vi "CAN自动测试.vi"(10 "选择?":bool) -> ()   [LabVIEW 2010]
uses:
  全局量/试验配置信息.vi
  全局量/自动测试结果.vi
panel:
  in  "同步_2":i32
  in  "同步_1":i32
  out "结束?":bool
  in  "CAN_4_4":u16
  in  "CAN_4_3":u16
  in  "CAN_4_2":u16
  in  "CAN_4_1":u16
  in  "CAN_3_4":u16
  in  "CAN_3_3":u16
  in  "CAN_3_2":u16
  in  "CAN_3_1":u16
  in  "CAN_2_4":u16
  in  "CAN_2_3":u16
  in  "CAN_2_2":u16
  in  "CAN_2_1":u16
  in  "CAN_1_4":u16
  in  "CAN_1_3":u16
  in  "CAN_1_2":u16
  in  "CAN_1_1":u16
  # "CAN1"
  # "CAN2"
  # "CAN3"
  # "CAN4"
  # "测试结论："
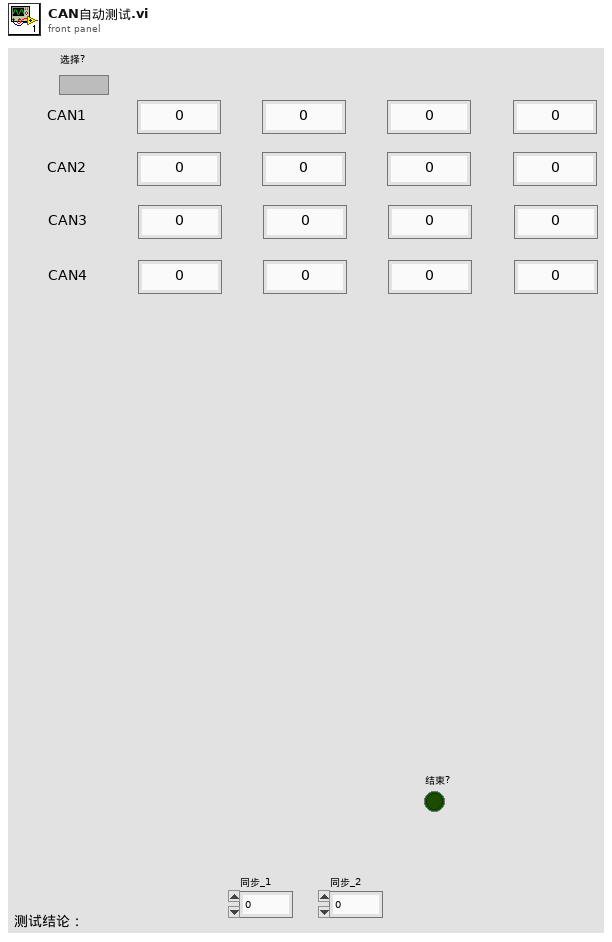
[diagram p1: front panel]
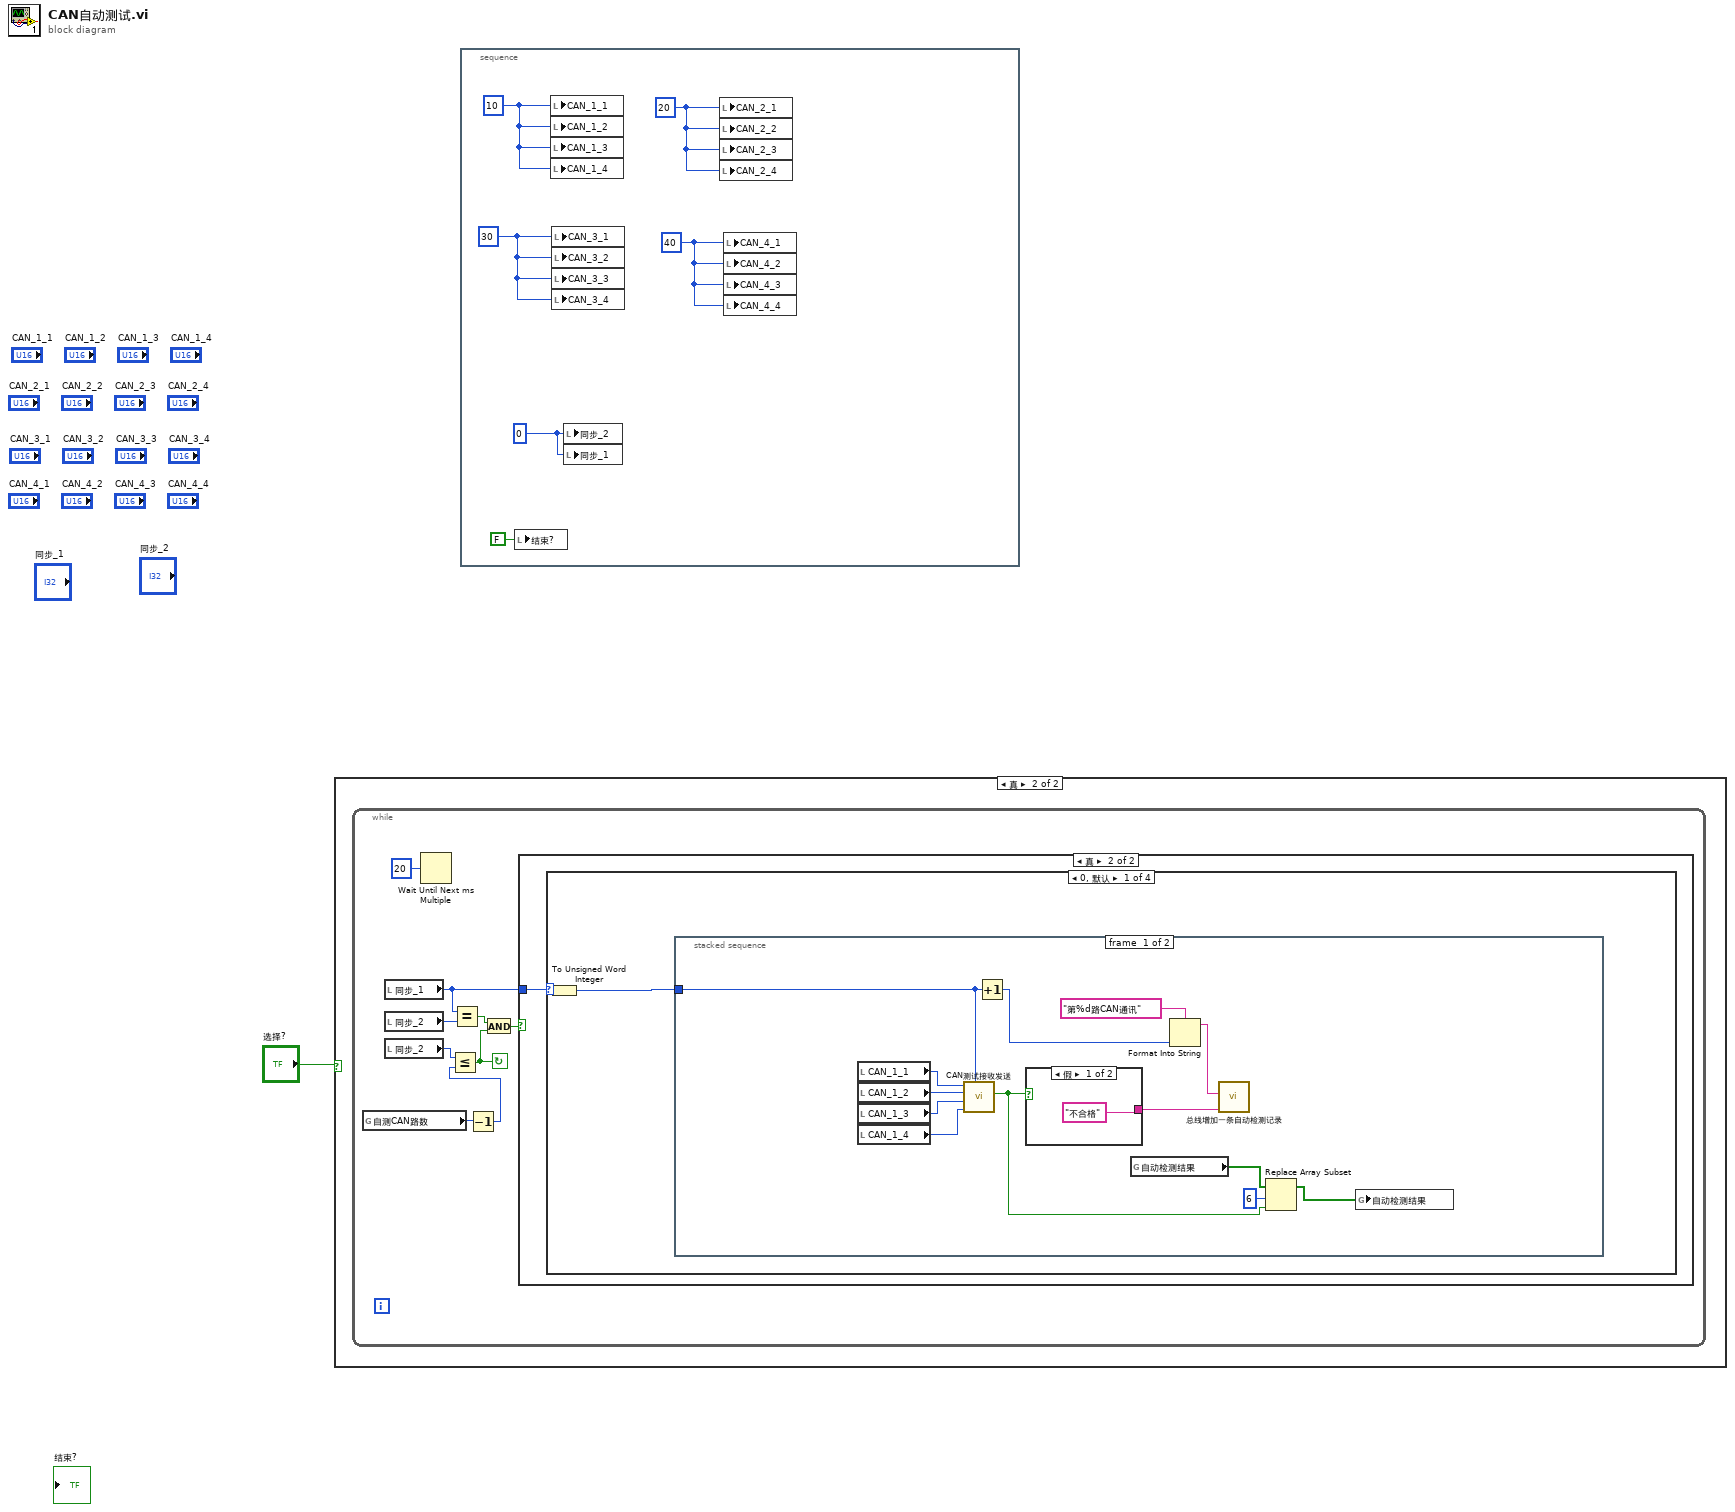
[diagram p0: block diagram]
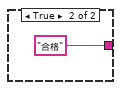
[diagram p4: hidden frame]
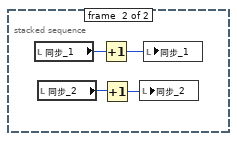
[diagram p5: hidden frame]
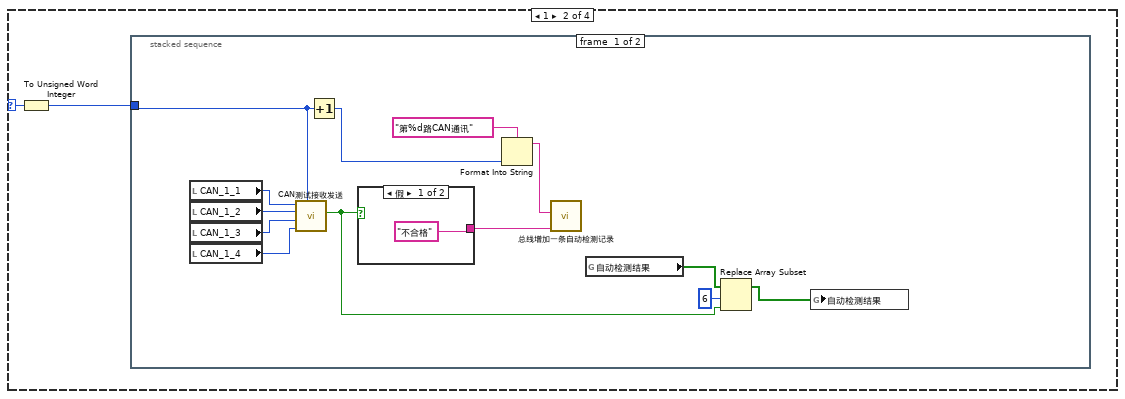
[diagram p6: hidden frame]
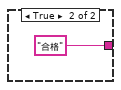
[diagram p7: hidden frame]
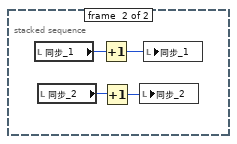
[diagram p8: hidden frame]
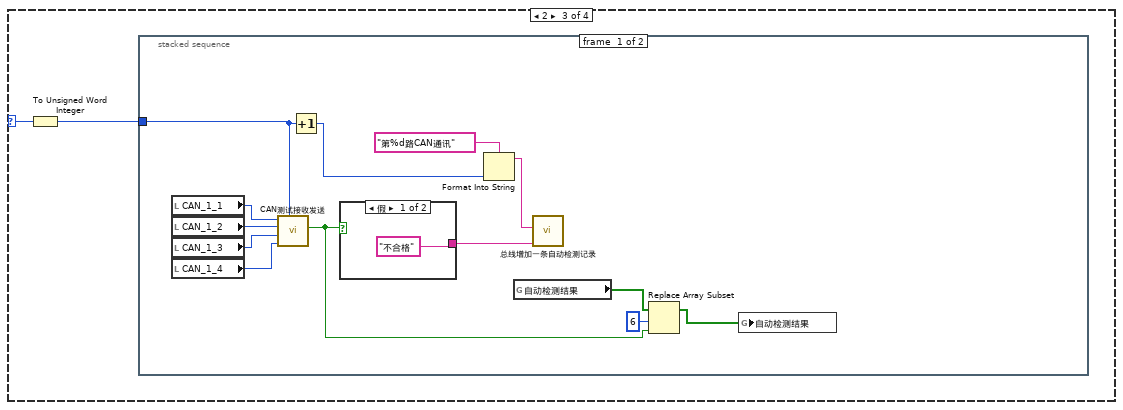
[diagram p9: hidden frame]
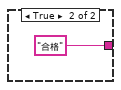
[diagram p10: hidden frame]
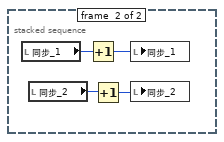
[diagram p11: hidden frame]
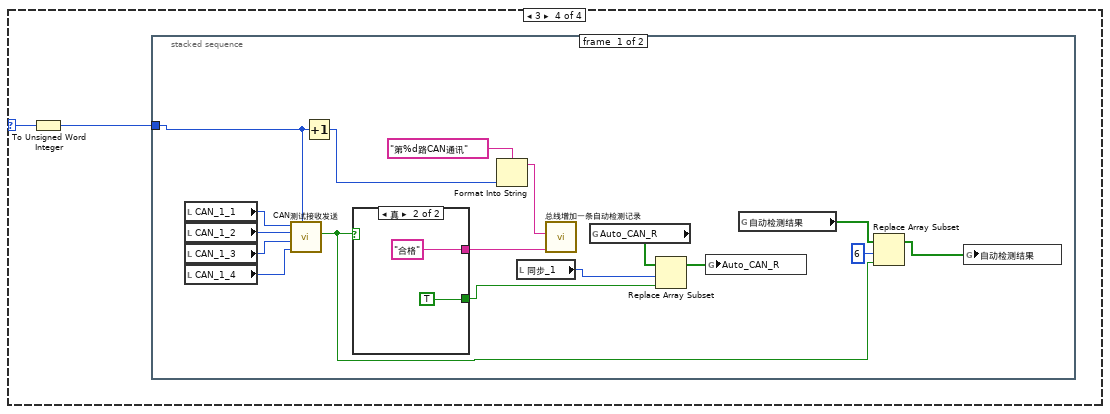
[diagram p12: hidden frame]
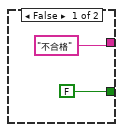
[diagram p13: hidden frame]
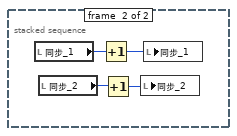
[diagram p14: hidden frame]
diagram:
  n1 = case shown="真" "选择?" {
    frame False {
    }
    frame True {
      n2 = while {
        stop <- w4 continue-if-true
        n3 = global read "试验配置信息.vi" "自测CAN路数"() -> (w3:i32)
        n4 = local read "同步_1"() -> (w10:i32)
        n5 = local read "同步_2"() -> (w7:i32)
        n6 = local read "同步_2"() -> (w9:i32)
        n7 = Wait Until Next ms Multiple(millisecond multiple=u32 20 ("毫秒倍数")) -> ()  [unwired: 1 out]
        n8 = Equal?(x=w10, y=w7) -> (x = y?=w5:bool)
        n9 = Decrement(x=w3) -> (x-1=w2:i32)
        n10 = Less Or Equal?(x=w9, y=w2) -> (x <= y?=w4:bool)
        n11 = And(x=w5, y=w4) -> (x .and. y?=w6:bool)
        n12 = case shown="真" w6 {
          tunnel: w10 -> [_ w11]
          frame False {
          }
          frame True {
            n13 = case shown="0, 默认" w11 {
              selector: w11 -> [w12 w34 w55 w76]
              frame 0, Default {
                n14 = To Unsigned Word Integer(number=w12) -> (unsigned 16bit integer=w13:u16)
                n15 = stacked-sequence {
                  tunnel: w13 -> [w22 _]
                  frame #0 {
                    n16 = local read "CAN_1_1"() -> (w23:u16)
                    n17 = local read "CAN_1_2"() -> (w24:u16)
                    n18 = local read "CAN_1_3"() -> (w25:u16)
                    n19 = local read "CAN_1_4"() -> (w26:u16)
                    n20 = call "CAN测试接收发送.vi"("Order"=w22, "data_4"=w26, "data_3"=w25, "data_2"=w24, "data_1"=w23) -> ("成功？"=w14:bool)  [unwired: 5 in, 1 out]
                    n21 = Increment(x=w22) -> (x+1=w20:u16)
                    n22 = case shown="假" w14 {
                      tunnel: ["不合格" "合格"] -> w18
                      frame False {
                      }
                      frame True {
                      }
                    }
                    n23 = global read "试验配置信息.vi" "自动检测结果"() -> (w15:bool[])
                    n24 = Format Into String(format string="第%d路CAN通讯", w20) -> (resulting string=w19:string)  [unwired: 2 in, 1 out]
                    n25 = call "总线增加一条自动检测记录.vi"("测试结果"=w18, "测试内容"=w19) -> ()  [unwired: 10 in]
                    n26 = Replace Array Subset(array=w15, new element=w14, index=6 ("索引")) -> (w16:bool[])
                    n27 = global write "试验配置信息.vi" "自动检测结果"(w16) -> ()
                  }
                  frame #1 {
                    n28 = local read "同步_1"() -> (w31:i32)
                    n29 = local read "同步_2"() -> (w29:i32)
                    n30 = Increment(x=w31) -> (x+1=w32:i32)
                    n31 = Increment(x=w29) -> (x+1=w30:i32)
                    n32 = local write "同步_2"(w30) -> ()
                    n33 = local write "同步_1"(w32) -> ()
                  }
                }
              }
              frame 1 {
                n34 = To Unsigned Word Integer(number=w34) -> (unsigned 16bit integer=w33:u16)
                n35 = stacked-sequence {
                  tunnel: w33 -> [w39 _]
                  frame #0 {
                    n36 = local read "CAN_1_1"() -> (w44:u16)
                    n37 = local read "CAN_1_2"() -> (w45:u16)
                    n38 = local read "CAN_1_3"() -> (w46:u16)
                    n39 = local read "CAN_1_4"() -> (w47:u16)
                    n40 = call "CAN测试接收发送.vi"("Order"=w39, "data_4"=w47, "data_3"=w46, "data_2"=w45, "data_1"=w44) -> ("成功？"=w35:bool)  [unwired: 5 in, 1 out]
                    n41 = Increment(x=w39) -> (x+1=w42:u16)
                    n42 = case shown="假" w35 {
                      tunnel: ["不合格" "合格"] -> w40
                      frame False {
                      }
                      frame True {
                      }
                    }
                    n43 = Format Into String(format string="第%d路CAN通讯", w42) -> (resulting string=w41:string)  [unwired: 2 in, 1 out]
                    n44 = call "总线增加一条自动检测记录.vi"("测试结果"=w40, "测试内容"=w41) -> ()  [unwired: 10 in]
                    n45 = global read "试验配置信息.vi" "自动检测结果"() -> (w36:bool[])
                    n46 = Replace Array Subset(array=w36, new element=w35, index=6 ("索引")) -> (w37:bool[])
                    n47 = global write "试验配置信息.vi" "自动检测结果"(w37) -> ()
                  }
                  frame #1 {
                    n48 = local read "同步_1"() -> (w52:i32)
                    n49 = local read "同步_2"() -> (w51:i32)
                    n50 = Increment(x=w52) -> (x+1=w53:i32)
                    n51 = Increment(x=w51) -> (x+1=w50:i32)
                    n52 = local write "同步_2"(w50) -> ()
                    n53 = local write "同步_1"(w53) -> ()
                  }
                }
              }
              frame 2 {
                n54 = To Unsigned Word Integer(number=w55) -> (unsigned 16bit integer=w54:u16)
                n55 = stacked-sequence {
                  tunnel: w54 -> [w60 _]
                  frame #0 {
                    n56 = local read "CAN_1_1"() -> (w65:u16)
                    n57 = local read "CAN_1_2"() -> (w66:u16)
                    n58 = local read "CAN_1_3"() -> (w67:u16)
                    n59 = local read "CAN_1_4"() -> (w68:u16)
                    n60 = call "CAN测试接收发送.vi"("Order"=w60, "data_4"=w68, "data_3"=w67, "data_2"=w66, "data_1"=w65) -> ("成功？"=w56:bool)  [unwired: 5 in, 1 out]
                    n61 = Increment(x=w60) -> (x+1=w63:u16)
                    n62 = case shown="假" w56 {
                      tunnel: ["不合格" "合格"] -> w61
                      frame False {
                      }
                      frame True {
                      }
                    }
                    n63 = Format Into String(format string="第%d路CAN通讯", w63) -> (resulting string=w62:string)  [unwired: 2 in, 1 out]
                    n64 = global read "试验配置信息.vi" "自动检测结果"() -> (w57:bool[])
                    n65 = call "总线增加一条自动检测记录.vi"("测试结果"=w61, "测试内容"=w62) -> ()  [unwired: 10 in]
                    n66 = Replace Array Subset(array=w57, new element=w56, index=6 ("索引")) -> (w58:bool[])
                    n67 = global write "试验配置信息.vi" "自动检测结果"(w58) -> ()
                  }
                  frame #1 {
                    n68 = local read "同步_1"() -> (w73:i32)
                    n69 = local read "同步_2"() -> (w71:i32)
                    n70 = Increment(x=w73) -> (x+1=w74:i32)
                    n71 = Increment(x=w71) -> (x+1=w72:i32)
                    n72 = local write "同步_1"(w74) -> ()
                    n73 = local write "同步_2"(w72) -> ()
                  }
                }
              }
              frame 3 {
                n74 = To Unsigned Word Integer(number=w76) -> (unsigned 16bit integer=w75:u16)
                n75 = stacked-sequence {
                  tunnel: w75 -> [w85 _]
                  frame #0 {
                    n76 = local read "CAN_1_1"() -> (w90:u16)
                    n77 = local read "CAN_1_2"() -> (w91:u16)
                    n78 = local read "CAN_1_3"() -> (w92:u16)
                    n79 = local read "CAN_1_4"() -> (w93:u16)
                    n80 = call "CAN测试接收发送.vi"("Order"=w85, "data_4"=w93, "data_3"=w92, "data_2"=w91, "data_1"=w90) -> ("成功？"=w77:bool)  [unwired: 5 in, 1 out]
                    n81 = Increment(x=w85) -> (x+1=w88:u16)
                    n82 = case shown="真" w77 {
                      tunnel: ["不合格" "合格"] -> w86
                      tunnel: [FALSE TRUE] -> w81
                      frame False {
                      }
                      frame True {
                      }
                    }
                    n83 = Format Into String(format string="第%d路CAN通讯", w88) -> (resulting string=w87:string)  [unwired: 2 in, 1 out]
                    n84 = local read "同步_1"() -> (w82:i32)
                    n85 = call "总线增加一条自动检测记录.vi"("测试结果"=w86, "测试内容"=w87) -> ()  [unwired: 10 in]
                    n86 = global read "自动测试结果.vi" "Auto_CAN_R"() -> (w84:bool[])
                    n87 = Replace Array Subset(array=w84, new element=w81, index=w82) -> (w83:bool[])
                    n88 = global write "自动测试结果.vi" "Auto_CAN_R"(w83) -> ()
                    n89 = global read "试验配置信息.vi" "自动检测结果"() -> (w78:bool[])
                    n90 = Replace Array Subset(array=w78, new element=w77, index=6 ("索引")) -> (w79:bool[])
                    n91 = global write "试验配置信息.vi" "自动检测结果"(w79) -> ()
                  }
                  frame #1 {
                    n92 = local read "同步_1"() -> (w101:i32)
                    n93 = local read "同步_2"() -> (w98:i32)
                    n94 = Increment(x=w101) -> (x+1=w100:i32)
                    n95 = Increment(x=w98) -> (x+1=w99:i32)
                    n96 = local write "同步_2"(w99) -> ()
                    n97 = local write "同步_1"(w100) -> ()
                  }
                }
              }
            }
          }
        }
      }
    }
  }
  n98 = stacked-sequence {
    frame #0 {
      w102 = u16 30 ("CAN_R_3_1")
      w103 = u16 40 ("CAN_R_4_1")
      w104 = u16 20 ("CAN_R_2_1")
      w105 = u16 10 ("CAN_R_1_1")
      w106 = 0 ("同步_2")
      n99 = local write "结束?"(FALSE ("结束?")) -> ()
      n100 = local write "CAN_1_1"(w105) -> ()
      n101 = local write "CAN_1_2"(w105) -> ()
      n102 = local write "CAN_1_3"(w105) -> ()
      n103 = local write "CAN_1_4"(w105) -> ()
      n104 = local write "CAN_3_1"(w102) -> ()
      n105 = local write "CAN_3_2"(w102) -> ()
      n106 = local write "CAN_3_3"(w102) -> ()
      n107 = local write "CAN_3_4"(w102) -> ()
      n108 = local write "同步_2"(w106) -> ()
      n109 = local write "同步_1"(w106) -> ()
      n110 = local write "CAN_2_1"(w104) -> ()
      n111 = local write "CAN_2_2"(w104) -> ()
      n112 = local write "CAN_2_3"(w104) -> ()
      n113 = local write "CAN_2_4"(w104) -> ()
      n114 = local write "CAN_4_1"(w103) -> ()
      n115 = local write "CAN_4_2"(w103) -> ()
      n116 = local write "CAN_4_3"(w103) -> ()
      n117 = local write "CAN_4_4"(w103) -> ()
    }
  }
